vi "LM Display Cntrl.vi"() -> ()   [LabVIEW 2010]
panel:
  out "Meas Illum":dbl format="%#_4g"
  in  "Backlight":bool
  out "error out":errorcluster {"code" format="%.0x"}
  in  "error in (no error)":errorcluster
  in  "VISA Session":refnum<visa-resource-name>
  # "LM Display Cntrl"
  # "nW/cm^2"
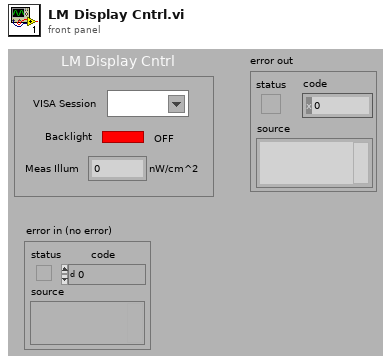
[diagram p1: front panel]
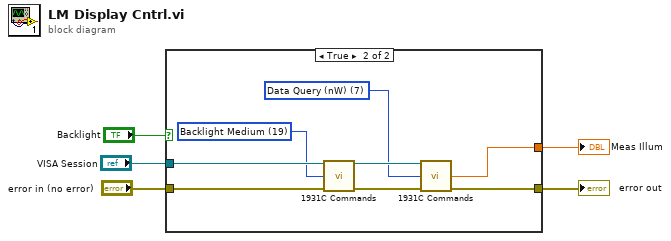
[diagram p0: block diagram]
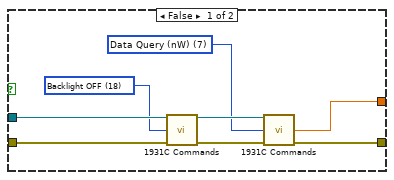
[diagram p2: hidden frame]
diagram:
  n1 = case shown="True" "Backlight" {
    tunnel: "VISA Session" -> [w13 w21]
    tunnel: "error in (no error)" -> [w12 w20]
    tunnel: [w9 w17] -> w2
    tunnel: [w6 w14] -> w1
    frame False {
      w7 = u16 7 items=["Attenuator OFF", "Attenuator ON", "Attenuator Query", "Beep OFF", "Beep ON", "Beep Query", "Clear Status Reg", "Data Query (nW)", "Echo OFF", "Echo ON", "Echo Query", "No Filter", "Analog Filter", "Digital FIlter", "Filter Query", "Hold", "Go", "Go Query", "Backlight OFF", "Backlight Medium", "Backlight High", "Backlight Query", "Set Dsplay Screen 0", "Set Display Screen 1", "Display Screen Query", "Mode DC Continuous", "Mode DC Single", "Mode Integrate", "Identification", "Auto Range", "Auto Range Query", "Signal Range 0", "Signal Range 1", "Signal Range 2", "Signal Range 3", "Signal Range 4", "Signal Range 5", "Signal Range 6", "Signal Range Query", "Store Reference", "Units W", "Units W/cm2", "Units dBm", "Units Joules", "Units Query", "Set Wavelength", "Wavelength Querry", "Mode Pesk-to-Peak Cont.", "Mode Peak-to-Peak Sing.", "Mode Query"] ("Command")
      w11 = u16 18 items=["Attenuator OFF", "Attenuator ON", "Attenuator Query", "Beep OFF", "Beep ON", "Beep Query", "Clear Status Reg", "Data Query (nW)", "Echo OFF", "Echo ON", "Echo Query", "No Filter", "Analog Filter", "Digital FIlter", "Filter Query", "Hold", "Go", "Go Query", "Backlight OFF", "Backlight Medium", "Backlight High", "Backlight Query", "Set Dsplay Screen 0", "Set Display Screen 1", "Display Screen Query", "Mode DC Continuous", "Mode DC Single", "Mode Integrate", "Identification", "Auto Range", "Auto Range Query", "Signal Range 0", "Signal Range 1", "Signal Range 2", "Signal Range 3", "Signal Range 4", "Signal Range 5", "Signal Range 6", "Signal Range Query", "Store Reference", "Units W", "Units W/cm2", "Units dBm", "Units Joules", "Units Query", "Set Wavelength", "Wavelength Querry", "Mode Pesk-to-Peak Cont.", "Mode Peak-to-Peak Sing.", "Mode Query"] ("Command")
      n2 = call "1931C Commands.vi"("Instrument Resource Name"=w13, "Command"=w11, "error in (no error)"=w12) -> ("VISA resource name out"=w8:refnum<visa-resource-name>, "error out"=w10:errorcluster)  [unwired: 8 in, 3 out]
      n3 = call "1931C Commands.vi"("Instrument Resource Name"=w8, "Command"=w7, "error in (no error)"=w10) -> ("LM Response"=w6:dbl, "error out"=w9:errorcluster)  [unwired: 8 in, 3 out]
    }
    frame True {
      w15 = u16 7 items=["Attenuator OFF", "Attenuator ON", "Attenuator Query", "Beep OFF", "Beep ON", "Beep Query", "Clear Status Reg", "Data Query (nW)", "Echo OFF", "Echo ON", "Echo Query", "No Filter", "Analog Filter", "Digital FIlter", "Filter Query", "Hold", "Go", "Go Query", "Backlight OFF", "Backlight Medium", "Backlight High", "Backlight Query", "Set Dsplay Screen 0", "Set Display Screen 1", "Display Screen Query", "Mode DC Continuous", "Mode DC Single", "Mode Integrate", "Identification", "Auto Range", "Auto Range Query", "Signal Range 0", "Signal Range 1", "Signal Range 2", "Signal Range 3", "Signal Range 4", "Signal Range 5", "Signal Range 6", "Signal Range Query", "Store Reference", "Units W", "Units W/cm2", "Units dBm", "Units Joules", "Units Query", "Set Wavelength", "Wavelength Querry", "Mode Pesk-to-Peak Cont.", "Mode Peak-to-Peak Sing.", "Mode Query"] ("Command")
      w19 = u16 19 items=["Attenuator OFF", "Attenuator ON", "Attenuator Query", "Beep OFF", "Beep ON", "Beep Query", "Clear Status Reg", "Data Query (nW)", "Echo OFF", "Echo ON", "Echo Query", "No Filter", "Analog Filter", "Digital FIlter", "Filter Query", "Hold", "Go", "Go Query", "Backlight OFF", "Backlight Medium", "Backlight High", "Backlight Query", "Set Dsplay Screen 0", "Set Display Screen 1", "Display Screen Query", "Mode DC Continuous", "Mode DC Single", "Mode Integrate", "Identification", "Auto Range", "Auto Range Query", "Signal Range 0", "Signal Range 1", "Signal Range 2", "Signal Range 3", "Signal Range 4", "Signal Range 5", "Signal Range 6", "Signal Range Query", "Store Reference", "Units W", "Units W/cm2", "Units dBm", "Units Joules", "Units Query", "Set Wavelength", "Wavelength Querry", "Mode Pesk-to-Peak Cont.", "Mode Peak-to-Peak Sing.", "Mode Query"] ("Command")
      n4 = call "1931C Commands.vi"("Instrument Resource Name"=w21, "Command"=w19, "error in (no error)"=w20) -> ("VISA resource name out"=w16:refnum<visa-resource-name>, "error out"=w18:errorcluster)  [unwired: 8 in, 3 out]
      n5 = call "1931C Commands.vi"("Instrument Resource Name"=w16, "Command"=w15, "error in (no error)"=w18) -> ("LM Response"=w14:dbl, "error out"=w17:errorcluster)  [unwired: 8 in, 3 out]
    }
  }
  "error out" <- w2
  "Meas Illum" <- w1
